vi "AOTF_frequency_amplitude _Initialization_final.vi"() -> ()   [LabVIEW 2009]
uses:
  <userlib>/AotfLibrary/AotfLibrary.lvlib
panel:
  out "concatenated string 9":string
  out "concatenated string 8":string
  out "concatenated string 2":string
  out "concatenated string":string
  out "concatenated string 6":string
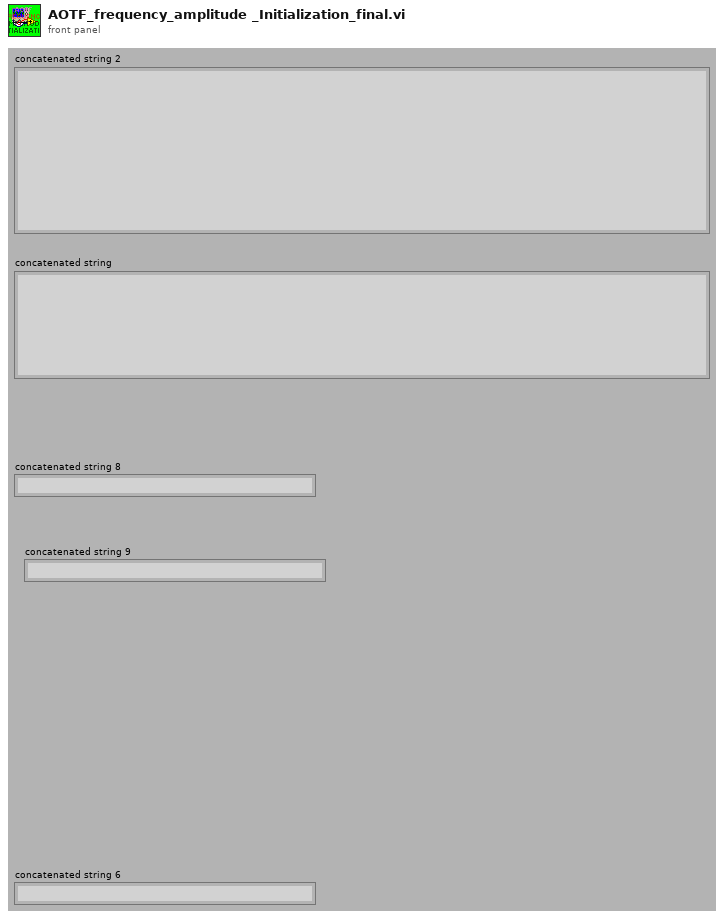
[diagram p1: front panel]
types:
  T1 = typedef "AOTFSettings.ctt" = cluster{"Laser 1 Output Channel":tag, "AOTF  1 Output Voltage":dbl, "Laser 2 Output Channel":tag, "AOTF  2 Output Voltage":dbl, "Laser 3 Output Channel":tag, "AOTF  3 Output Voltage":dbl, "Pixel per Cycle":u16, "Time per Cycle  / ms":dbl, "Laser 4 Output Channel":tag, "AOTF  4 Output Voltage":dbl, "Laser 5 Output Channel":tag, "AOTF 5 Output Voltage ":dbl, "Laser 6 Output Channel":tag, "AOTF  6 Output Voltage ":dbl, "Laser 7 Output Channel":tag, "AOTF 7 Output Voltage ":dbl, "Laser 8 Output Channel":tag, "AOTF  8 Output Voltage ":dbl, "AOTF  1 Frequency":dbl, "AOTF  2 Frequency":dbl, "AOTF  3  Frequency":dbl, "AOTF  4 Frequency":dbl, "AOTF 5 Frequency":dbl, "AOTF  6 Frequency":dbl, "AOTF 7  Frequency":dbl, "AOTF  8 Frequency":dbl, "AOTF  1 Amplitude":dbl, "AOTF  2 Amplitude":dbl, "AOTF  3  Amplitude":dbl, "AOTF  4 Amplitude":dbl, "AOTF 5 Amplitude":dbl, "AOTF  6 Amplitude":dbl, "AOTF 7 Amplitude  ":dbl, "AOTF  8 Amplitude":dbl}
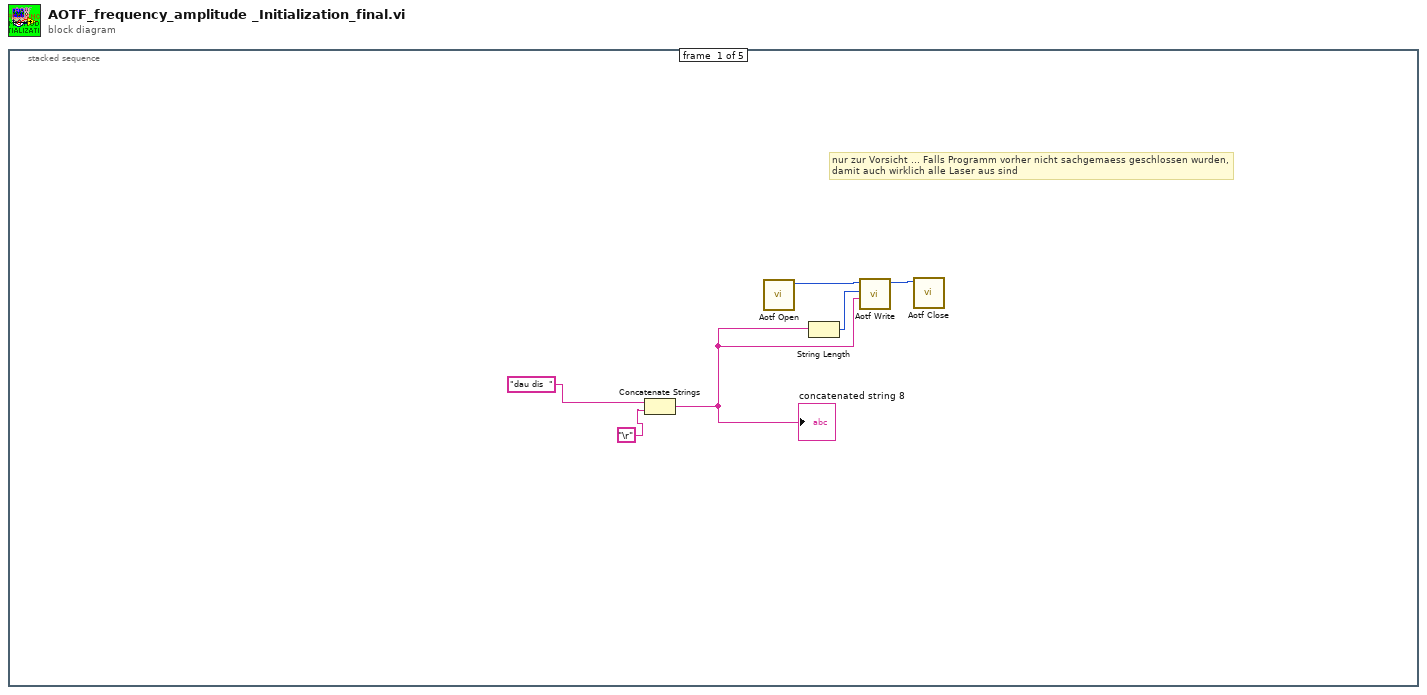
[diagram p0: block diagram]
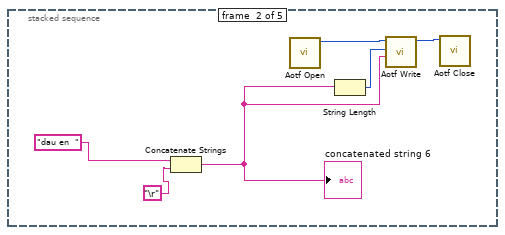
[diagram p2: hidden frame]
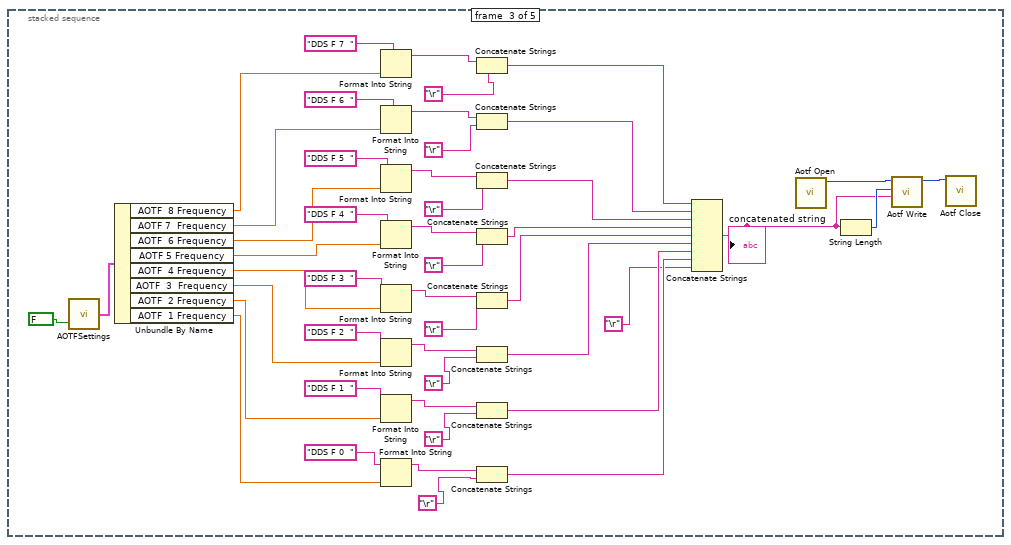
[diagram p3: hidden frame]
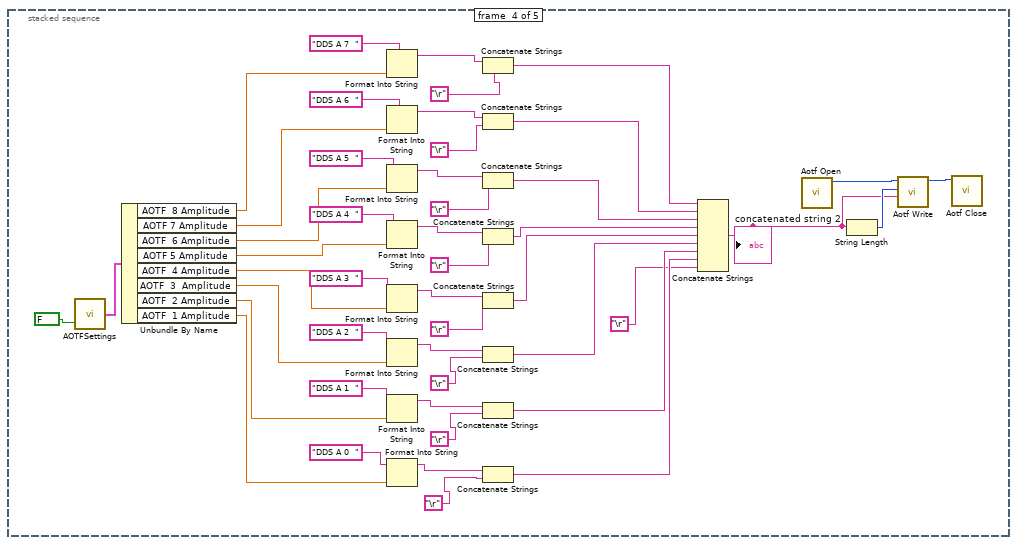
[diagram p4: hidden frame]
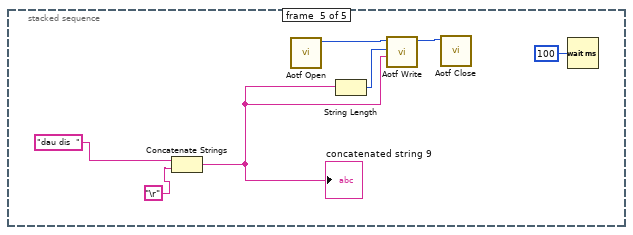
[diagram p5: hidden frame]
diagram:
  n1 = stacked-sequence {
    frame #0 {
      # "nur zur Vorsicht ... Falls Programm vorher nicht sachgemaess geschlossen wurden, \ndamit auch wirklich alle Laser aus sind"
      n2 = Concatenate Strings("dau dis  " ("string"), "\r") -> (w2:string)
      "concatenated string 8" <- w2
      n3 = call <userlib>:"Aotf Open.vi"() -> ("function return"=w5:u32)  [unwired: 11 in]
      n4 = String Length(string=w2) -> (length=w4:i32)
      n5 = call <userlib>:"Aotf Write.vi"("pData"=w2, "uiLength"=w4, "hAotfController"=w5) -> ("hAotfController out"=w6:u32)  [unwired: 7 in, 1 out]
      n6 = call <userlib>:"Aotf Close.vi"("hAotfController"=w6) -> ()  [unwired: 9 in, 2 out]
    }
    frame #1 {
      n7 = Concatenate Strings("dau en  " ("string"), "\r") -> (w8:string)
      "concatenated string 6" <- w8
      n8 = call <userlib>:"Aotf Open.vi"() -> ("function return"=w11:u32)  [unwired: 11 in]
      n9 = String Length(string=w8) -> (length=w10:i32)
      n10 = call <userlib>:"Aotf Write.vi"("pData"=w8, "uiLength"=w10, "hAotfController"=w11) -> ("hAotfController out"=w12:u32)  [unwired: 7 in, 1 out]
      n11 = call <userlib>:"Aotf Close.vi"("hAotfController"=w12) -> ()  [unwired: 9 in, 2 out]
    }
    frame #2 {
      n12 = call "AOTFSettings.vi"("Get/Set"=FALSE) -> ("AOTF Setting (Output)"=w57:T1)  [unwired: 1 in]
      n13 = Unbundle By Name(w57) -> ("AOTF  8 Frequency"=w34:dbl, "AOTF 7  Frequency"=w33:dbl, "AOTF  6 Frequency"=w32:dbl, "AOTF 5 Frequency"=w31:dbl, "AOTF  4 Frequency"=w27:dbl, "AOTF  3  Frequency"=w28:dbl, "AOTF  2 Frequency"=w29:dbl, "AOTF  1 Frequency"=w30:dbl)
      n14 = Format Into String(initial string="DDS F 7  " ("string"), w34) -> (resulting string=w37:string)  [unwired: 2 in, 1 out]
      n15 = Format Into String(initial string="DDS F 6  " ("string"), w33) -> (resulting string=w39:string)  [unwired: 2 in, 1 out]
      n16 = Format Into String(initial string="DDS F 5  " ("string"), w32) -> (resulting string=w42:string)  [unwired: 2 in, 1 out]
      n17 = Format Into String(initial string="DDS F 4  " ("string"), w31) -> (resulting string=w45:string)  [unwired: 2 in, 1 out]
      n18 = Format Into String(initial string="DDS F 3  " ("string"), w27) -> (resulting string=w48:string)  [unwired: 2 in, 1 out]
      n19 = Format Into String(initial string="DDS F 2  " ("string"), w28) -> (resulting string=w51:string)  [unwired: 2 in, 1 out]
      n20 = Format Into String(initial string="DDS F 1  " ("string"), w29) -> (resulting string=w54:string)  [unwired: 2 in, 1 out]
      n21 = Format Into String(initial string="DDS F 0  " ("string"), w30) -> (resulting string=w59:string)  [unwired: 2 in, 1 out]
      n22 = Concatenate Strings(w37, "\r") -> (w22:string)
      n23 = Concatenate Strings(w39, "\r") -> (w23:string)
      n24 = Concatenate Strings(w42, "\r") -> (w24:string)
      n25 = Concatenate Strings(w45, "\r") -> (w25:string)
      n26 = Concatenate Strings(w48, "\r") -> (w21:string)
      n27 = Concatenate Strings(w51, "\r") -> (w19:string)
      n28 = Concatenate Strings(w54, "\r") -> (w18:string)
      n29 = Concatenate Strings(w59, "\r") -> (w20:string)
      n30 = Concatenate Strings(w22, w23, w24, w25, w21, w19, w18, w20, "\r") -> (w13:string)
      "concatenated string" <- w13
      n31 = call <userlib>:"Aotf Open.vi"() -> ("function return"=w15:u32)  [unwired: 11 in]
      n32 = String Length(string=w13) -> (length=w16:i32)
      n33 = call <userlib>:"Aotf Write.vi"("pData"=w13, "uiLength"=w16, "hAotfController"=w15) -> ("hAotfController out"=w14:u32)  [unwired: 7 in, 1 out]
      n34 = call <userlib>:"Aotf Close.vi"("hAotfController"=w14) -> ()  [unwired: 9 in, 2 out]
    }
    frame #3 {
      n35 = call "AOTFSettings.vi"("Get/Set"=FALSE) -> ("AOTF Setting (Output)"=w104:T1)  [unwired: 1 in]
      n36 = Unbundle By Name(w104) -> ("AOTF  8 Amplitude"=w81:dbl, "AOTF 7 Amplitude"=w80:dbl, "AOTF  6 Amplitude"=w79:dbl, "AOTF 5 Amplitude"=w78:dbl, "AOTF  4 Amplitude"=w74:dbl, "AOTF  3  Amplitude"=w75:dbl, "AOTF  2 Amplitude"=w76:dbl, "AOTF  1 Amplitude"=w77:dbl)
      n37 = Format Into String(initial string="DDS A 7  " ("string"), w81) -> (resulting string=w84:string)  [unwired: 2 in, 1 out]
      n38 = Format Into String(initial string="DDS A 6  " ("string"), w80) -> (resulting string=w86:string)  [unwired: 2 in, 1 out]
      n39 = Format Into String(initial string="DDS A 5  " ("string"), w79) -> (resulting string=w89:string)  [unwired: 2 in, 1 out]
      n40 = Format Into String(initial string="DDS A 4  " ("string"), w78) -> (resulting string=w92:string)  [unwired: 2 in, 1 out]
      n41 = Format Into String(initial string="DDS A 3  " ("string"), w74) -> (resulting string=w95:string)  [unwired: 2 in, 1 out]
      n42 = Format Into String(initial string="DDS A 2  " ("string"), w75) -> (resulting string=w98:string)  [unwired: 2 in, 1 out]
      n43 = Format Into String(initial string="DDS A 1  " ("string"), w76) -> (resulting string=w101:string)  [unwired: 2 in, 1 out]
      n44 = Format Into String(initial string="DDS A 0  " ("string"), w77) -> (resulting string=w106:string)  [unwired: 2 in, 1 out]
      n45 = Concatenate Strings(w84, "\r") -> (w69:string)
      n46 = Concatenate Strings(w86, "\r") -> (w70:string)
      n47 = Concatenate Strings(w89, "\r") -> (w71:string)
      n48 = Concatenate Strings(w92, "\r") -> (w72:string)
      n49 = Concatenate Strings(w95, "\r") -> (w68:string)
      n50 = Concatenate Strings(w98, "\r") -> (w66:string)
      n51 = Concatenate Strings(w101, "\r") -> (w65:string)
      n52 = Concatenate Strings(w106, "\r") -> (w67:string)
      n53 = Concatenate Strings(w69, w70, w71, w72, w68, w66, w65, w67, "\r") -> (w60:string)
      "concatenated string 2" <- w60
      n54 = call <userlib>:"Aotf Open.vi"() -> ("function return"=w62:u32)  [unwired: 11 in]
      n55 = String Length(string=w60) -> (length=w63:i32)
      n56 = call <userlib>:"Aotf Write.vi"("pData"=w60, "uiLength"=w63, "hAotfController"=w62) -> ("hAotfController out"=w61:u32)  [unwired: 7 in, 1 out]
      n57 = call <userlib>:"Aotf Close.vi"("hAotfController"=w61) -> ()  [unwired: 9 in, 2 out]
    }
    frame #4 {
      n58 = Concatenate Strings("dau dis  " ("string"), "\r") -> (w108:string)
      "concatenated string 9" <- w108
      n59 = call <userlib>:"Aotf Open.vi"() -> ("function return"=w111:u32)  [unwired: 11 in]
      n60 = String Length(string=w108) -> (length=w110:i32)
      n61 = call <userlib>:"Aotf Write.vi"("pData"=w108, "uiLength"=w110, "hAotfController"=w111) -> ("hAotfController out"=w112:u32)  [unwired: 7 in, 1 out]
      n62 = call <userlib>:"Aotf Close.vi"("hAotfController"=w112) -> ()  [unwired: 9 in, 2 out]
      n63 = Wait (ms)(milliseconds to wait=u32 100) -> ()  [unwired: 1 out]
    }
  }
